vi "SW_Gen_Get_Initial_picture_Scaling_and_Cage_size_DAQmx.vi"(7 "Input cluster of parameters":T3={"Cage diameter, mm"=180, "Starting angle MIDFIELD"=0, "Starting angle BORDER"=0, "Radius, mm CENTER"=30, "Radius, mm MIDFIELD"=60, "N segments MIDFIELD"=4, "N segments BORDER"=8, "R-gap, mm"=0.0, "Bridge swap"=FALSE, "Bridge H. offset"=0.0, "Bridge V. offset"=0.0, "Twisted neck"=FALSE, "Alt. magn. orientation"=FALSE, "Sensor board size"=enum."Small"} {"Cage diameter, mm" scale=0.0..340.0}, 8 "Error In":errorcluster, 9 "Scale factor for outer display radius display":dbl=0.95 format="%#_13g", 10 "Background color":u32(colorbox)=13816530, 11 "Draw Area Size":T4={"Width"=480, "Height"=480}) -> (0 "Error Out":errorcluster, 1 "Width of the borders combined out":cluster{"Width":i32, "Height":i32}, 2 "Image geometrical and scaling parameters":T2, 3 "Background Image":T1(plugin-control))   [LabVIEW 2018, in "Tracker.lvlib"]
uses:
  Tracker.lvlib
  Controls/CTL_Draw_Area_Size.ctl
  Controls/CTL_Segmented_plot_parameters.ctl
  Controls/CTL_Image_Geometrical_and_scaling_parameters.ctl
panel:
  in  "Width of the borders combined":cluster{"Width":i32, "Height":i32}
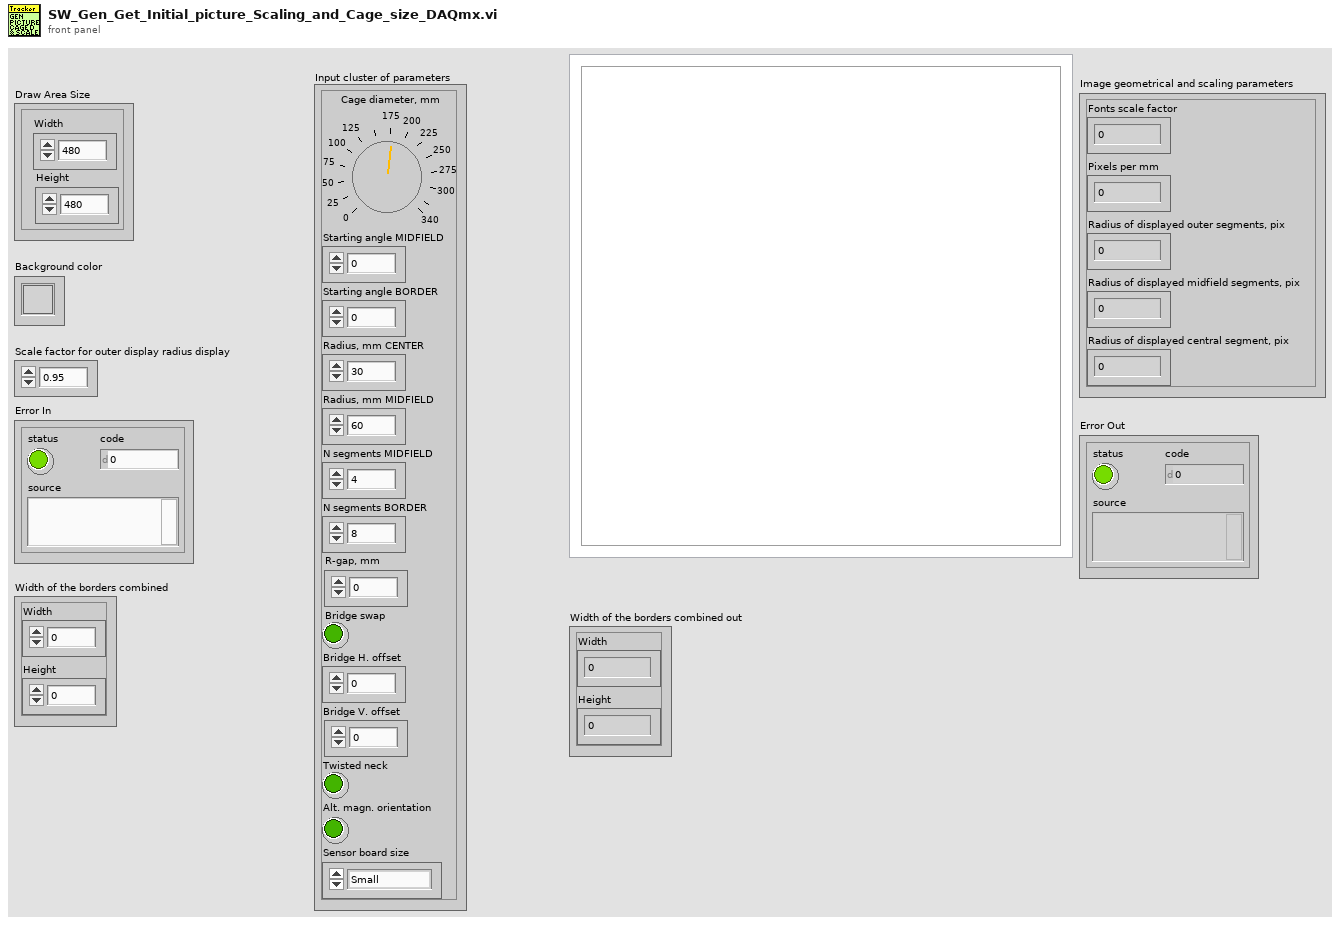
[diagram p1: front panel]
types:
  T1 = typedef "IMAQ Image.ctl" = refnum<image>
  T2 = typedef "Tracker.lvlib/CTL_Image_Geometrical_and_scaling_parameters.ctl" = cluster{"Fonts scale factor":dbl, "Pixels per mm":dbl, "Radius of displayed outer segments, pix":dbl, "Radius of displayed midfield segments, pix":dbl, "Radius of displayed central segment, pix":dbl}
  T3 = typedef "Tracker.lvlib/CTL_Segmented_plot_parameters.ctl" = cluster{"Cage diameter, mm":u16, "Starting angle MIDFIELD":i16, "Starting angle BORDER":i16, "Radius, mm CENTER":u16, "Radius, mm MIDFIELD":u16, "N segments MIDFIELD":u8, "N segments BORDER":u8, "R-gap, mm":sgl, "Bridge swap":bool, "Bridge H. offset":sgl, "Bridge V. offset":sgl, "Twisted neck":bool, "Alt. magn. orientation":bool, "Sensor board size":enum16{"Small", "Large"}}
  T4 = typedef "Tracker.lvlib/CTL_Draw_Area_Size.ctl" = cluster{"Width":i32, "Height":i32}
  T5 = cluster{"Left":i32, "Top":i32, "Right":i32, "Bottom":i32}
  T6 = typedef "Image Type" = u32
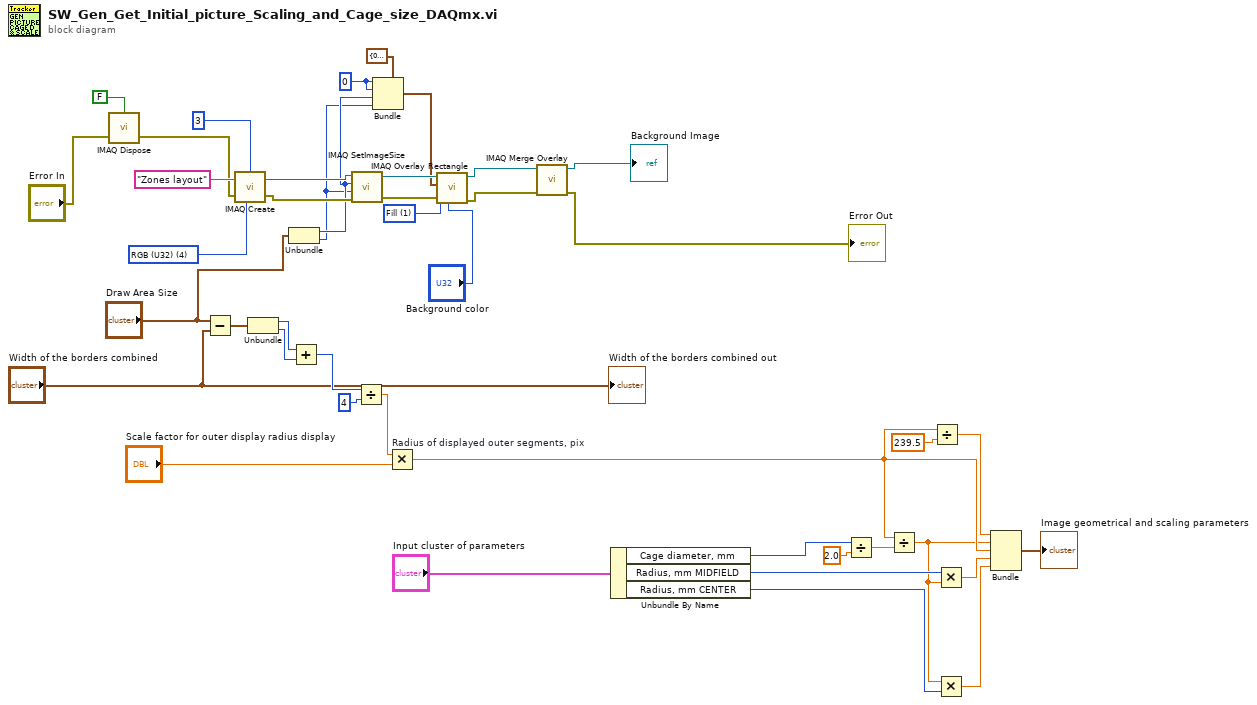
[diagram p0: block diagram]
diagram:
  w9 = 0 ("Left")
  w14 = u32 1 items=["Frame", "Fill", "Highlight"] ("Drawing Mode (Frame)")
  w20 = T6 4 items=["Grayscale (U8)", "Grayscale (I16)", "Grayscale (SGL)", "Complex (CSG)", "RGB (U32)", "HSL (U32)", "RGB (U64)", "Grayscale (U16)"] ("Image Type")
  n1 = call "IMAQ Dispose"("All Images? (No)"=FALSE, "error in (no error)"="Error In") -> ("error out"=w2:errorcluster)  [unwired: 4 in]
  n2 = Subtract(x="Draw Area Size", y="Width of the borders combined") -> (x-y=w35:T4)
  n3 = call "IMAQ Create"("Border Size"=3, "Image Name"="Zones layout", "Image Type"=w20, "error in (no error)"=w2) -> ("New Image"=w18:T1, "error out"=w19:errorcluster)  [unwired: 1 in]
  n4 = Unbundle(w35) -> ("Width"=w42:i32, "Height"=w43:i32)
  n5 = Unbundle("Draw Area Size") -> ("Width"=w11:i32, "Height"=w10:i32)
  n6 = Add(x=w42, y=w43) -> (x+y=w41:i32)
  n7 = call "IMAQ SetImageSize"("error in (no error)"=w19, "Y Resolution"=w10, "X Resolution"=w11, "Image"=w18) -> ("error out"=w17:errorcluster, "Image Out"=w16:T1)  [unwired: 1 in]
  n8 = Divide(x=w41, y=u32 4) -> (x/y=w38:dbl)
  n9 = Bundle(cluster=T5 {"Left"=0, "Top"=0, "Right"=480, "Bottom"=480} ("Rectangle"), "Left"=w9, "Top"=w9, "Right"=w11, "Bottom"=w10) -> (w12:T5)
  n10 = Multiply "Radius of displayed outer segments, pix"(x=w38, y="Scale factor for outer display radius display") -> (x*y=w29:dbl)
  n11 = call "IMAQ Overlay Rectangle"("Color"="Background color", "error in (no error)"=w17, "Drawing Mode (Frame)"=w14, "Rectangle"=w12, "Image"=w16) -> ("error out"=w7:errorcluster, "Image Out"=w8:T1)  [unwired: 5 in]
  n12 = call "IMAQ Merge Overlay"("error in (no error)"=w7, "Image Src"=w8) -> ("error out"=→"Error Out":errorcluster, "Image Dst Out"=→"Background Image":T1)  [unwired: 8 in]
  n13 = Unbundle By Name("Input cluster of parameters") -> ("Cage diameter, mm"=w31:u16, "Radius, mm MIDFIELD"=w28:u16, "Radius, mm CENTER"=w26:u16)
  n14 = Divide(x=w31, y=2.0) -> (x/y=w33:dbl)
  n15 = Divide(x=w29, y=w33) -> (x/y=w27:dbl)
  n16 = Divide(x=w29, y=239.5) -> (x/y=w30:dbl)
  n17 = Multiply(x=w28, y=w27) -> (x*y=w25:dbl)
  n18 = Multiply(x=w27, y=w26) -> (x*y=w24:dbl)
  n19 = Bundle(w30, w27, w29, w25, w24) -> (→"Image geometrical and scaling parameters":cluster{dbl, dbl, dbl, dbl, dbl})  [unwired: 1 in]
  "Width of the borders combined out" <- "Width of the borders combined"
